vi "UpdateIcon.vi"(8 "error in (no error)":errorcluster, 10 "Text":T1={"Line 1 text"="Example", "Line 2 text"="Test", "Line 3 text"="", "Line 4 text"=""}, 11 "VI Refnum in":refnum<vi>) -> (0 "error out":errorcluster, 3 "VI Refnum out":refnum<vi>)   [LabVIEW 2017]
doc: "This example reads the current icon of a VI and updates it with an entirely new icon which primarily focuses on the Template Layer."
uses:
  <vilib>/LabVIEW Icon API/API_Text.ctl
  <vilib>/LabVIEW Icon API/LabVIEW Icon API.lvlib
  <vilib>/addons/InsightCM/MessageBus/CodeGen/MessageGen.lvlib
panel:
  out "New VI Icon":picture
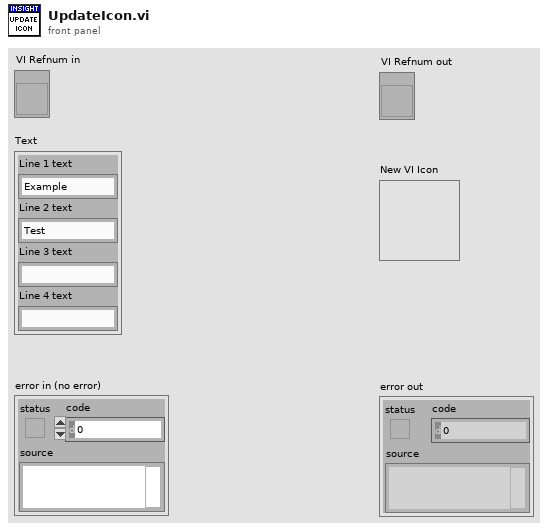
[diagram p1: front panel]
types:
  T1 = typedef "LabVIEW Icon API.lvlib/API_Text.ctl" = cluster{"Line 1 text":string, "Line 2 text":string, "Line 3 text":string, "Line 4 text":string}
  T2 = typedef "imagedata.ctl" = cluster{"image type":i32, "image depth":i32, "image":u8[], "mask":u8[], "colors":u32[], "Rectangle":cluster{"left":i16, "top":i16, "right":i16, "bottom":i16}}
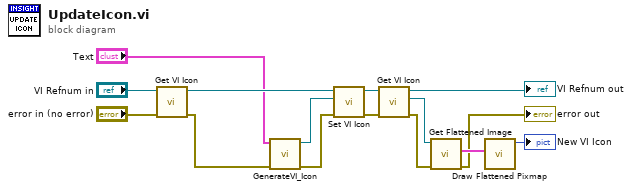
[diagram p0: block diagram]
diagram:
  n1 = call <vilib>:"Get VI Icon.vi"("error in (no error)"="error in (no error)", "VI Refnum in"="VI Refnum in") -> ("error out"=w3:errorcluster, "VI Refnum out"=w15:refnum<vi>)  [unwired: 7 in, 1 out]
  n2 = call <vilib>:"GenerateVI_Icon.vi"("error in (no error)"=w3, "Text"="Text") -> ("error out"=w14:errorcluster, "Icon.lvlclass out"=w13:refnum<class "Icon.lvclass">)  [unwired: 7 in, 1 out]
  n3 = call <vilib>:"Set VI Icon.vi"("error in (no error)"=w14, "Icon"=w13, "VI Refnum in"=w15) -> ("error out"=w10:errorcluster, "VI Refnum out"=w9:refnum<vi>)  [unwired: 7 in]
  n4 = call <vilib>:"Get VI Icon.vi"("error in (no error)"=w10, "VI Refnum in"=w9) -> ("error out"=w8:errorcluster, "Icon"=w7:refnum<class "Icon.lvclass">, "VI Refnum out"=→"VI Refnum out":refnum<vi>)  [unwired: 7 in]
  n5 = call <vilib>:"Get Flattened Image.vi"("error in (no error)"=w8, "lv_icon.lvlib:Icon.lvclass in"=w7) -> ("error out"=→"error out":errorcluster, "Color Image"=w11:T2)  [unwired: 6 in, 2 out]
  n6 = call <vilib>:"Draw Flattened Pixmap.vi"("image data"=w11) -> ("new picture"=→"New VI Icon":picture)  [unwired: 8 in]
